vi "RT_DynamicPressure.vi"(8 "V (m/s)":dbl[](array[numeric]), 9 "i":i32, 10 "V_wind [m/s]":dbl[][](array[numeric]), 11 "h (m)":dbl format="%#_13g") -> (0 "Patm (Pa)":dbl, 1 "air flow velocity [m/s]":dbl, 2 "Temp [K]":dbl, 3 "Pdin":dbl)   [LabVIEW 2011]
uses:
  <vilib>/Analysis/_algsub.llb/Vector Norm Type.ctl
  <vilib>/Analysis/_algsub.llb/Real Vector Norm.vi
  <vilib>/Analysis/NI_AALPro.lvlib
panel:
  out "rho (kg/m^3)":dbl
  out "p (Pa)":dbl
  out "T(ºC)":dbl
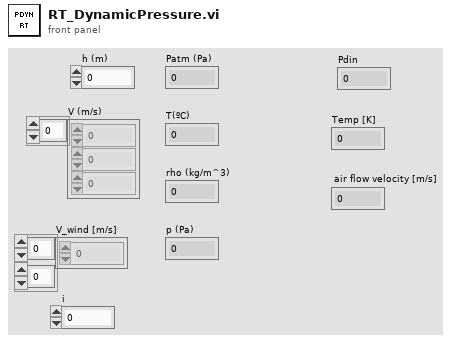
[diagram p1: front panel]
types:
  T1 = typedef "NI_AALPro.lvlib/Vector Norm Type.ctl" = u16
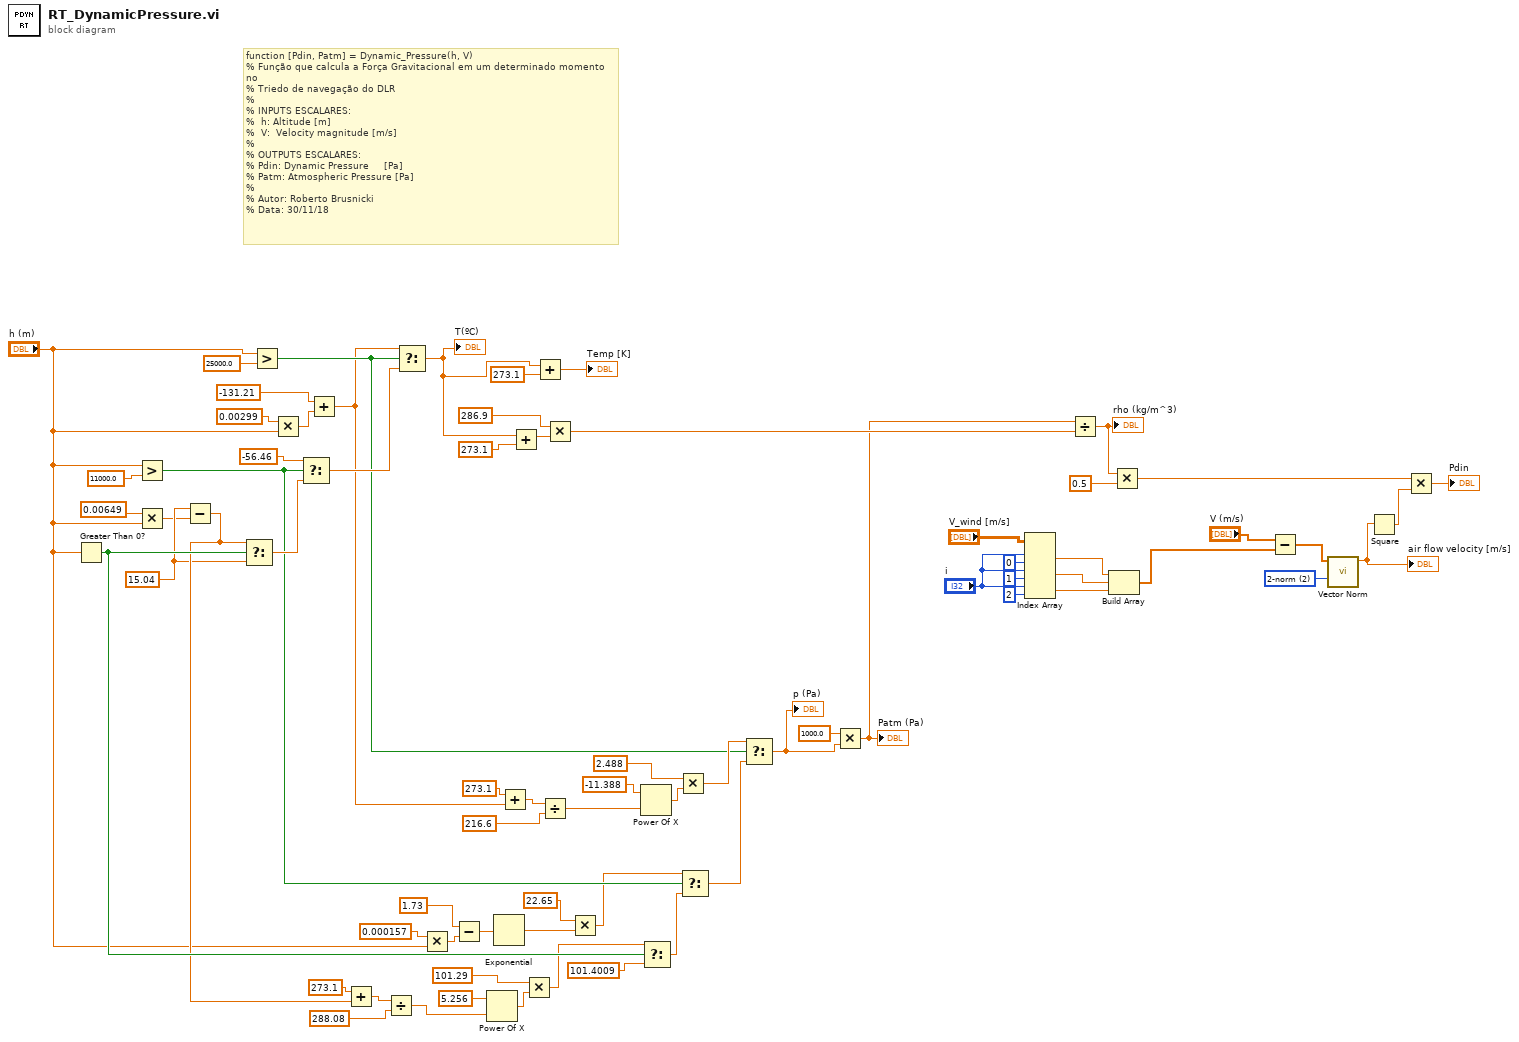
[diagram p0: block diagram]
diagram:
  w21 = T1 2 items=["1-norm"=1, "2-norm"=2, "Inf-norm"=3, "-Inf-norm"=4, "User Defined"=5] ("norm type")
  w49 = 15.04 ("x")
  # "function [Pdin, Patm] = Dynamic_Pressure(h, V)\n% Função que calcula a Força Gravitacional em um determinado momento no \n% Triedo de navegação do DLR\n%\n% INPUTS ESCALARES:\n%  h: Altitude [m]\n%  V:  Velocity magnitude [m/s]\n%\n% OUTPUTS ESCALARES:\n% Pdin: Dynamic Pressure     [Pa]\n% Patm: Atmospheric Pressure [Pa]\n%\n% Autor: Roberto Brusnicki\n% Data: 30/11/18"
  n1 = Greater Than 0?(x="h (m)") -> (x > 0?=w58:bool)
  n2 = Greater?(x="h (m)", y=11000.0) -> (0:w43:bool)
  n3 = Multiply(x=0.00649 ("y"), y="h (m)") -> (x*y=w45:dbl)
  n4 = Subtract(x=w49, y=w45) -> (x-y=w56:dbl)
  n5 = Select(t=w56, s=w58, f=w49) -> (s? t:f=w48:dbl)
  n6 = Greater?(x="h (m)", y=25000.0) -> (0:w26:bool)
  n7 = Multiply(x=0.00299 ("y"), y="h (m)") -> (x*y=w24:dbl)
  n8 = Select(t=-56.46, s=w43, f=w48) -> (s? t:f=w34:dbl)
  n9 = Add(x=-131.21 ("y"), y=w24) -> (x+y=w13:dbl)
  n10 = Add(x=273.1 ("y"), y=w56) -> (x+y=w54:dbl)
  n11 = Divide(x=w54, y=288.08) -> (x/y=w16:dbl)
  n12 = Select(t=w13, s=w26, f=w34) -> (s? t:f=w2:dbl)
  "T(ºC)" <- w2
  n13 = Multiply(x=0.000157 ("y"), y="h (m)") -> (x*y=w37:dbl)
  n14 = Subtract(x=1.73, y=w37) -> (x-y=w39:dbl)
  n15 = Power Of X(1:w16, 2:5.256 ("x")) -> (0:w51:dbl)
  n16 = Exponential(1:w39) -> (0:w40:dbl)
  n17 = Add(x=273.1 ("y"), y=w13) -> (x+y=w28:dbl)
  n18 = Add(x=w2, y=273.1) -> (x+y=w63:dbl)
  n19 = Multiply(x=101.29, y=w51) -> (x*y=w57:dbl)
  n20 = Add(x=w2, y=273.1) -> (x+y=→"Temp [K]":dbl)
  n21 = Divide(x=w28, y=216.6) -> (x/y=w18:dbl)
  n22 = Multiply(x=286.9, y=w63) -> (x*y=w66:dbl)
  n23 = Multiply(x=22.65, y=w40) -> (x*y=w42:dbl)
  n24 = Power Of X(1:w18, 2:-11.388 ("x")) -> (0:w35:dbl)
  n25 = Select(t=w57, s=w58, f=101.4009) -> (s? t:f=w50:dbl)
  n26 = Multiply(x=2.488, y=w35) -> (x*y=w31:dbl)
  n27 = Select(t=w42, s=w43, f=w50) -> (s? t:f=w44:dbl)
  n28 = Select(t=w31, s=w26, f=w44) -> (s? t:f=w60:dbl)
  "p (Pa)" <- w60
  n29 = Multiply(x=1000.0, y=w60) -> (x*y=w65:dbl)
  "Patm (Pa)" <- w65
  n30 = Index Array(array="V_wind [m/s]", index (row) #1="i", index (col) #1=0 ("disabled index (col)"), index (row) #2="i", index (col) #2=1 ("disabled index (col)"), index (row) #3="i", index (col) #3=2 ("disabled index (col)")) -> (element #1=w4:dbl, element #2=w7:dbl, element #3=w6:dbl)
  n31 = Divide(x=w65, y=w66) -> (x/y=w68:dbl)
  "rho (kg/m^3)" <- w68
  n32 = Build Array(w4, w7, w6) -> (w5:dbl[])
  n33 = Multiply(x=w68, y=0.5 ("x")) -> (x*y=w69:dbl)
  n34 = Subtract(x="V (m/s)", y=w5) -> (x-y=w14:dbl[])
  n35 = call-poly <vilib>:"Vector Norm.vi"("norm type"=w21, "Input Vector"=w14) -> ("norm"=w20:dbl)  [unwired: 8 in, 1 out]
  "air flow velocity [m/s]" <- w20
  n36 = Square(x=w20) -> (x^2=w70:dbl)
  n37 = Multiply(x=w69, y=w70) -> (x*y=→"Pdin":dbl)
